vi "Handle Message.vi"(8 "error in (no error)":errorcluster, 10 "Message":string, 11 "LabBOT in":refnum<class "LabBOT.lvclass">) -> (0 "error out":errorcluster, 2 "Close?":bool)   [LabVIEW 2020, in "Rover.lvlib" / "LabBOT.lvclass"]
uses:
  LabBOT.lvclass
  Control JSON.ctl
  LabBOT.lvclass/LabBOT.ctl
  Rover/Rover.lvclass
panel:
  out "Turn":dbl
  out "Drive":dbl
  out "cmdTurn":sgl(slide) scale=1.0..-1.0
  out "cmdDrive":sgl(slide) scale=-1.0..1.0
  in  "Turn Factor":dbl=1.0
  in  "Drive Factor":dbl=0.8
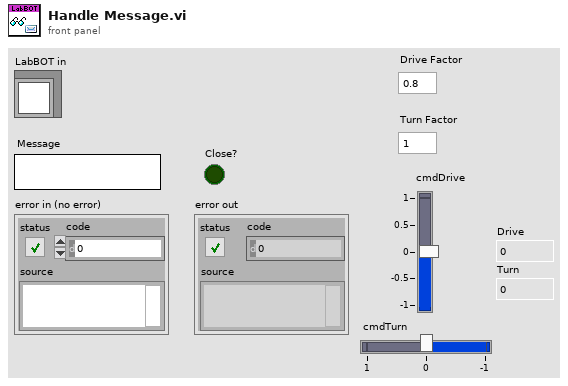
[diagram p1: front panel]
types:
  T1 = typedef "Rover.lvlib/LabBOT.lvclass/Control JSON.ctl" = cluster{"stop":bool, "drive":dbl, "turn":dbl}
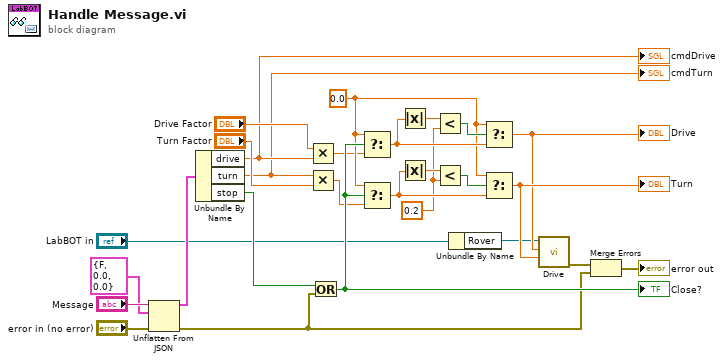
[diagram p0: block diagram]
diagram:
  w14 = 0.2 ("y")
  w13 = 0.0 ("t")
  n1 = Unflatten From JSON(JSON string="Message", type and defaults=T1 {"stop"=FALSE, "drive"=0.0, "turn"=0.0} ("Control JSON"), error in (no error)="error in (no error)") -> (value=w24:T1, error out=w9:errorcluster)  [unwired: 4 in]
  n2 = Unbundle By Name(w24) -> ("drive"=w4:dbl, "turn"=w3:dbl, "stop"=w23:bool)
  "cmdDrive" <- w4
  "cmdTurn" <- w3
  n3 = Multiply(x="Drive Factor", y=w4) -> (x*y=w6:dbl)
  n4 = Multiply(x=w3, y="Turn Factor") -> (x*y=w8:dbl)
  n5 = Or(x=w23, y=w9) -> (x .or. y?=w21:bool)
  "Close?" <- w21
  n6 = Select(t=w13, s=w21, f=w6) -> (s? t:f=w16:dbl)
  n7 = Select(t=w13, s=w21, f=w8) -> (s? t:f=w19:dbl)
  n8 = Absolute Value(x=w16) -> (abs(x)=w17:dbl)
  n9 = Absolute Value(x=w19) -> (abs(x)=w20:dbl)
  n10 = Less?(x=w17, y=w14) -> (x < y?=w15:bool)
  n11 = Less?(x=w20, y=w14) -> (x < y?=w18:bool)
  n12 = Unbundle By Name("LabBOT in") -> ("Rover"=w2:refnum<class "Rover.lvclass">)
  n13 = Select(t=w13, s=w15, f=w16) -> (s? t:f=w11:dbl)
  "Drive" <- w11
  n14 = Select(t=w13, s=w18, f=w19) -> (s? t:f=w12:dbl)
  "Turn" <- w12
  n15 = call "Drive.vi"("Turn"=w12, "Drive"=w11, "Rover in"=w2) -> ("error out"=w22:errorcluster)  [unwired: 7 in, 1 out]
  n16 = Merge Errors(w22, w9) -> (→"error out":errorcluster)
